vi "FGV Spectrometer.vi"(8 "entrée d'erreur (pas d'erreur)":errorcluster, 10 "FGV Spectro. Data":T1, 11 "Action":T2=enum."Initialisation") -> (0 "sortie d'erreur":errorcluster, 3 "Data out":T1)   [LabVIEW 2017]
doc: "Cett Variable globale fonctionnelle contrôle le Spectromètre. Il est possible alors de configurer plusieur évènements grace à l'énum \"Action\"\n\n1- Initialisation : crée un objet de classe wrapper permettant l'utilisation du spectromètre.\n2 - Get Device ID : Rend un tableau avec tous les numéro ID lié a chaque spectromètre branché sur le port usb de l'ordinateur\n3 - Select Device ID : Sélectionne le spectromètre qui va acquérir\n4 - Disable Calibration : Utilise la calibration d'usine\n5 - Enable calibration : utilise une calibration donnée se présentan sous la forme d'un tableau 1D\n6 - Set Averanging : Configuration du nombre de spectre moyenné lors de l'acquisition\n7 - Set Integrate Time : Configure le temps d'intégration\n8 - Get Spectrum : Réalise un spectre"
uses:
  Action Spectro.ctl
  FGV Spectro Data.ctl
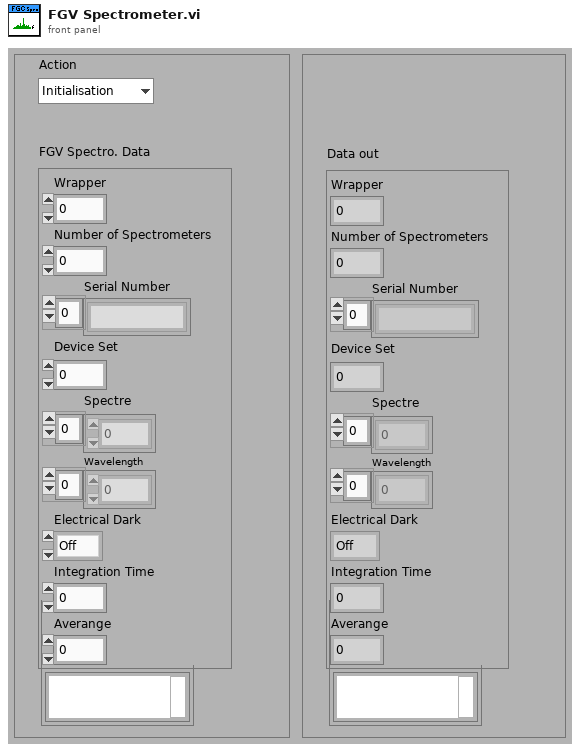
[diagram p1: front panel]
types:
  T1 = typedef "FGV Spectro Data.ctl" = cluster{"Wrapper":u32, "Number of Spectrometers":i32, "Serial Number":string[], "Device Set":i32, "Spectre":dbl[], "Wavelength":dbl[], "Electrical Dark":enum16{"Off", "On"}, "Integration Time":i32, "Averange":i32}
  T2 = typedef "Action Spectro.ctl" = enum16{"Connect", "Initialisation", "Set Device", "Set Intégration time", "Get integration Time", "Disable Noise Suppress", "Enable Noise Suppress", "Set Averange", "Get Spectrum", "Get WaveLength", "Abort", "Disconnect"}
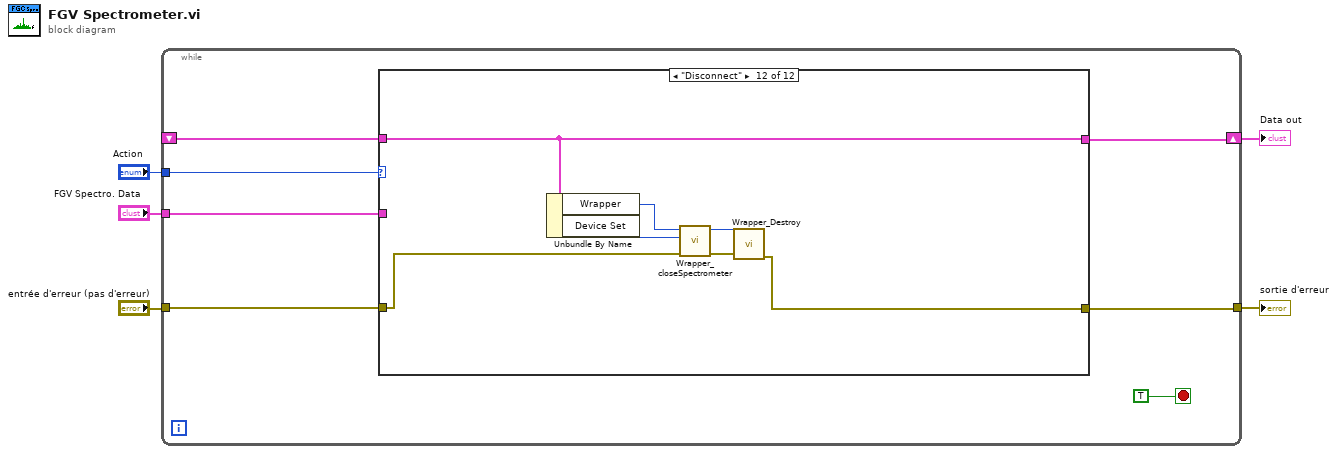
[diagram p0: block diagram]
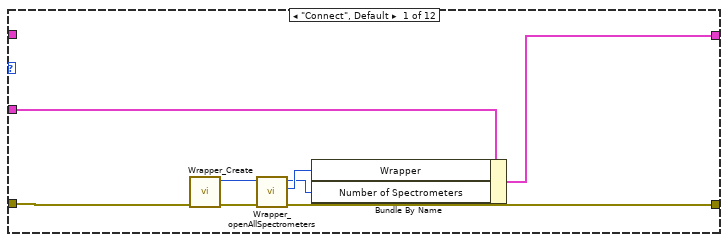
[diagram p2: hidden frame]
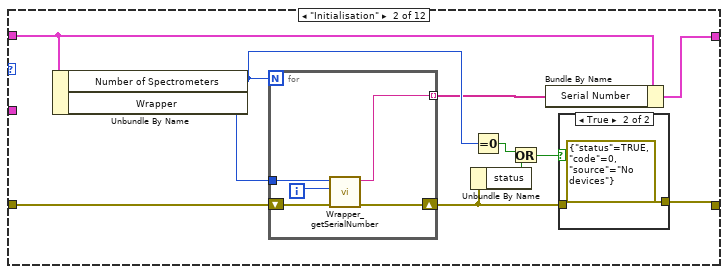
[diagram p3: hidden frame]
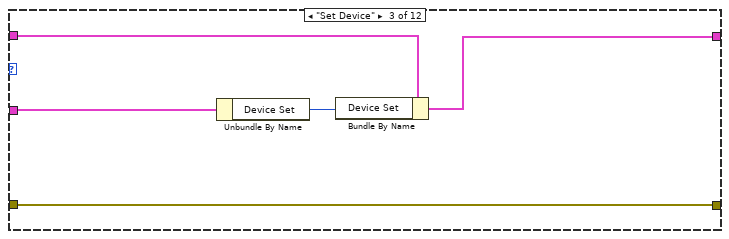
[diagram p5: hidden frame]
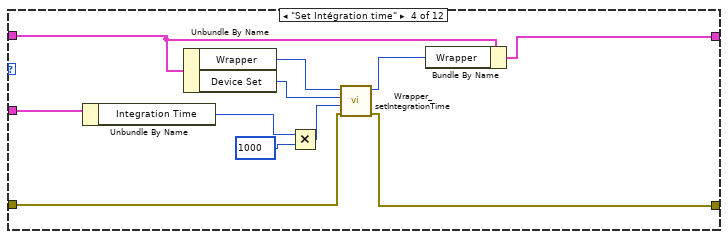
[diagram p6: hidden frame]
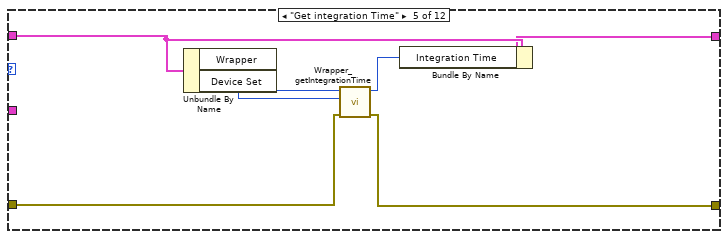
[diagram p7: hidden frame]
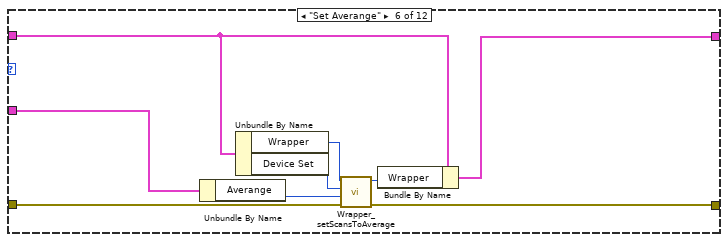
[diagram p8: hidden frame]
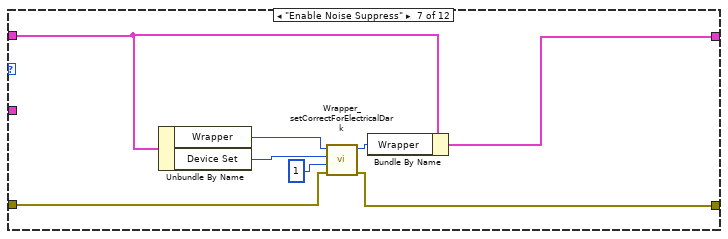
[diagram p9: hidden frame]
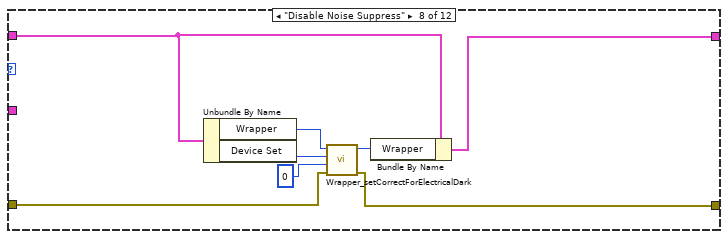
[diagram p10: hidden frame]
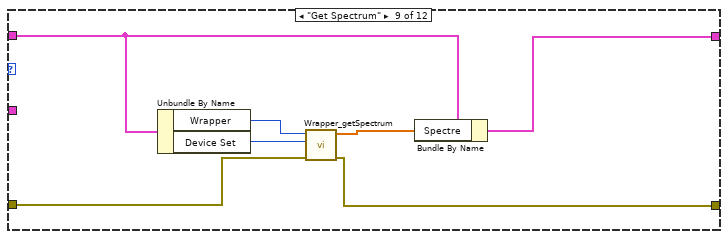
[diagram p11: hidden frame]
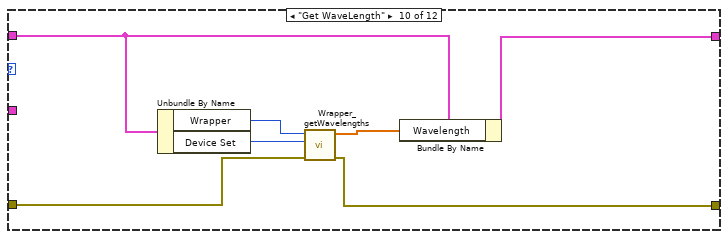
[diagram p12: hidden frame]
diagram:
  n1 = while {
    tunnel: "Action" -> [w9]
    tunnel: "entrée d'erreur (pas d'erreur)" -> [w11]
    tunnel: [w10] -> w4
    shift-right: [w7] -> w2
    shift-left: _ -> [w8]
    tunnel: "FGV Spectro. Data" -> [w6]
    stop <- TRUE stop-if-true
    n2 = case shown="\"Disconnect\"" w9 {
      tunnel: w11 -> [w18 w30 w43 w50 w57 w70 w75 w83 w89 w96 w102 w105]
      tunnel: [w17 w31 w43 w45 w56 w69 w74 w82 w88 w95 w102 w103] -> w10
      tunnel: [w14 w27 w39 w46 w60 w64 w71 w79 w87 w94 w101 w109] -> w7
      tunnel: w8 -> [_ w28 w41 w47 w61 w66 w72 w80 w93 w100 w101 w109]
      tunnel: w6 -> [w13 _ w42 w49 _ w63 _ _ _ _ _ _]
      frame "Connect", Default {
        n3 = call <userlib>:"Wrapper_Create.vi"("error in (no error)"=w18) -> ("error out"=w20:errorcluster, "Wrapper"=w19:u32)  [unwired: 9 in]
        n4 = call <userlib>:"Wrapper_openAllSpectrometers.vi"("error in (no error)"=w20, "Wrapper In"=w19) -> ("error out"=w17:errorcluster, "Wrapper Out"=w16:u32, "Number of Spectrometers"=w15:i32)  [unwired: 7 in]
        n5 = Bundle By Name(cluster=w13, "Wrapper"=w16, "Number of Spectrometers"=w15) -> (w14:T1)
      }
      frame "Initialisation" {
        n6 = Unbundle By Name(w28) -> ("Number of Spectrometers"=w29:i32, "Wrapper"=w26:u32)
        n7 = for {
          N: w29 -> [_]
          shift-right: [w34] -> w24
          shift-left: w30 -> [w38]
          tunnel: [w35] -> w25 mode=indexing
          tunnel: w26 -> [w36]
          i -> [w37]
          n8 = call <userlib>:"Wrapper_getSerialNumber.vi"("error in (no error)"=w38, "Index"=w37, "Wrapper"=w36) -> ("error out"=w34:errorcluster, "Serial Number"=w35:string)  [unwired: 7 in]
        }
        n9 = Unbundle By Name(w24) -> ("status"=w22:bool)
        n10 = Equal To 0?(x=w29) -> (x = 0?=w23:bool)
        n11 = Or(x=w23, y=w22) -> (x .or. y?=w21:bool)
        n12 = Bundle By Name(cluster=w28, "Serial Number"=w25) -> (w27:T1)
        n13 = case shown="True" w21 {
          tunnel: w24 -> [w32 _]
          tunnel: [w32 errorcluster {"status"=TRUE, "code"=0, "source"="No devices"} ("sortie d'erreur")] -> w31
          frame False {
          }
          frame True {
          }
        }
      }
      frame "Set Device" {
        n14 = Unbundle By Name(w42) -> ("Device Set"=w40:i32)
        n15 = Bundle By Name(cluster=w41, "Device Set"=w40) -> (w39:T1)
      }
      frame "Set Intégration time" {
        n16 = Unbundle By Name(w49) -> ("Integration Time"=w48:i32)
        n17 = Unbundle By Name(w47) -> ("Wrapper"=w51:u32, "Device Set"=w52:i32)
        n18 = Multiply(x=w48, y=1000) -> (x*y=w54:i32)
        n19 = call <userlib>:"Wrapper_setIntegrationTime.vi"("error in (no error)"=w50, "Integration Time"=w54, "Index"=w52, "Wrapper In"=w51) -> ("error out"=w45:errorcluster, "Wrapper Out"=w44:u32)  [unwired: 6 in]
        n20 = Bundle By Name(cluster=w47, "Wrapper"=w44) -> (w46:T1)
      }
      frame "Get integration Time" {
        n21 = Unbundle By Name(w61) -> ("Wrapper"=w59:u32, "Device Set"=w58:i32)
        n22 = call <userlib>:"Wrapper_getIntegrationTime.vi"("error in (no error)"=w57, "Index"=w58, "Wrapper"=w59) -> ("error out"=w56:errorcluster, "Integration Time"=w55:i32)  [unwired: 7 in]
        n23 = Bundle By Name(cluster=w61, "Integration Time"=w55) -> (w60:T1)
      }
      frame "Set Averange" {
        n24 = Unbundle By Name(w63) -> ("Averange"=w62:i32)
        n25 = Unbundle By Name(w66) -> ("Wrapper"=w68:u32, "Device Set"=w67:i32)
        n26 = call <userlib>:"Wrapper_setScansToAverage.vi"("error in (no error)"=w70, "Average"=w62, "Index"=w67, "Wrapper In"=w68) -> ("error out"=w69:errorcluster, "Wrapper Out"=w65:u32)  [unwired: 6 in]
        n27 = Bundle By Name(cluster=w66, "Wrapper"=w65) -> (w64:T1)
      }
      frame "Enable Noise Suppress" {
        n28 = Unbundle By Name(w72) -> ("Wrapper"=w78:u32, "Device Set"=w77:i32)
        n29 = call <userlib>:"Wrapper_setCorrectForElectricalDark.vi"("error in (no error)"=w75, "On/Off"=1, "Index"=w77, "Wrapper In"=w78) -> ("error out"=w74:errorcluster, "Wrapper Out"=w73:u32)  [unwired: 6 in]
        n30 = Bundle By Name(cluster=w72, "Wrapper"=w73) -> (w71:T1)
      }
      frame "Disable Noise Suppress" {
        n31 = Unbundle By Name(w80) -> ("Wrapper"=w86:u32, "Device Set"=w85:i32)
        n32 = call <userlib>:"Wrapper_setCorrectForElectricalDark.vi"("error in (no error)"=w83, "On/Off"=0, "Index"=w85, "Wrapper In"=w86) -> ("error out"=w82:errorcluster, "Wrapper Out"=w81:u32)  [unwired: 6 in]
        n33 = Bundle By Name(cluster=w80, "Wrapper"=w81) -> (w79:T1)
      }
      frame "Get Spectrum" {
        n34 = Unbundle By Name(w93) -> ("Wrapper"=w90:u32, "Device Set"=w91:i32)
        n35 = call <userlib>:"Wrapper_getSpectrum.vi"("error in (no error)"=w89, "Index"=w91, "Wrapper"=w90) -> ("error out"=w88:errorcluster, "Spectrum Values"=w92:dbl[])  [unwired: 6 in, 1 out]
        n36 = Bundle By Name(cluster=w93, "Spectre"=w92) -> (w87:T1)
      }
      frame "Get WaveLength" {
        n37 = Unbundle By Name(w100) -> ("Wrapper"=w99:u32, "Device Set"=w97:i32)
        n38 = call <userlib>:"Wrapper_getWavelengths.vi"("error in (no error)"=w96, "Index"=w97, "Wrapper"=w99) -> ("error out"=w95:errorcluster, "WL Values"=w98:dbl[])  [unwired: 6 in, 1 out]
        n39 = Bundle By Name(cluster=w100, "Wavelength"=w98) -> (w94:T1)
      }
      frame "Abort" {
      }
      frame "Disconnect" {
        n40 = Unbundle By Name(w109) -> ("Wrapper"=w108:u32, "Device Set"=w106:i32)
        n41 = call <userlib>:"Wrapper_closeSpectrometer.vi"("error in (no error)"=w105, "Index"=w106, "Wrapper In"=w108) -> ("error out"=w104:errorcluster, "Wrapper Out"=w107:u32)  [unwired: 7 in]
        n42 = call <userlib>:"Wrapper_Destroy.vi"("error in (no error)"=w104, "Wrapper"=w107) -> ("error out"=w103:errorcluster)  [unwired: 9 in]
      }
    }
  }
  "sortie d'erreur" <- w4
  "Data out" <- w2
